vi "Gantry_motion.vi"() -> ()   [LabVIEW 2016]
uses:
  Classes/Controllers/Motion/Copy of A3200 Folder/A3200.lvclass
  D:/INTT/V1/Classes/Controllers/Motion/Copy of Motion Folder/Motion.lvclass
  Classes/Controllers/Motion/Copy of Motion Folder/Motion.lvclass
panel:
  out "millisecond timer value":u32
  in  "Stop":bool
  in  "Z Speed":dbl=5.0 format="%#_13g"
  in  "Z":dbl=10.0 format="%#_13g"
  out "Gantry position":dbl[](array[numeric])
  in  "Speed":dbl=20.0
  in  "XY":dbl[](array[numeric])
  out "number of tasks excuted":i32
  in  "Z GO":bool
  in  "XY GO":bool
  in  "XYZ GO":bool
  in  "XYZTheta In":dbl[](array[numeric])=[600.0, 600.0, 0.0, 0.0]
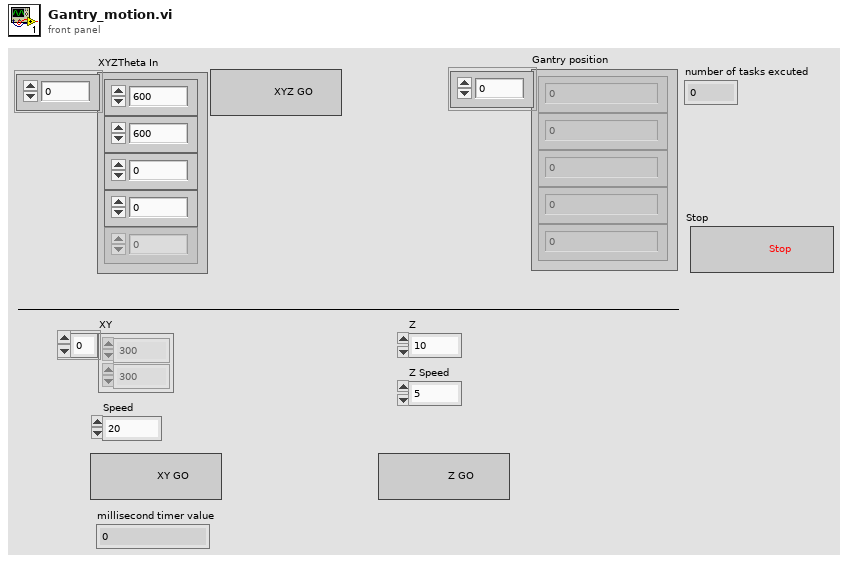
[diagram p1: front panel]
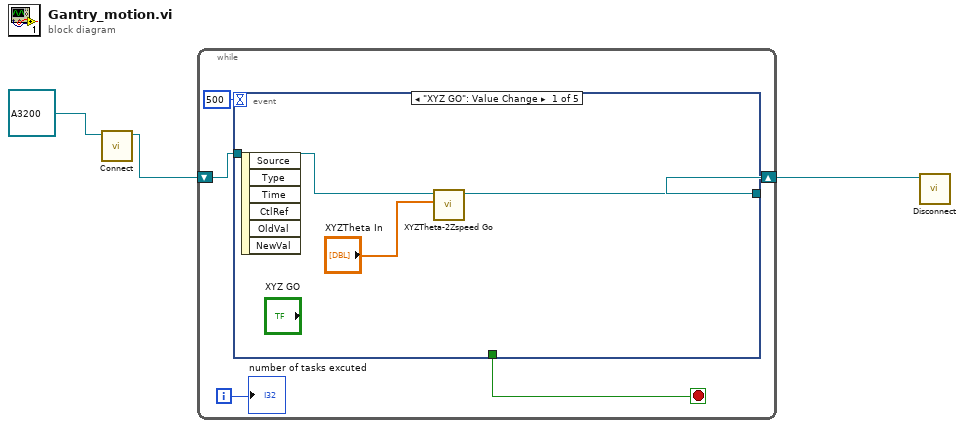
[diagram p0: block diagram]
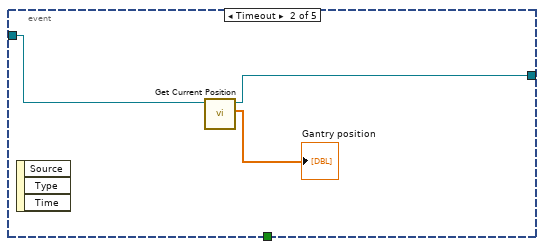
[diagram p2: hidden frame]
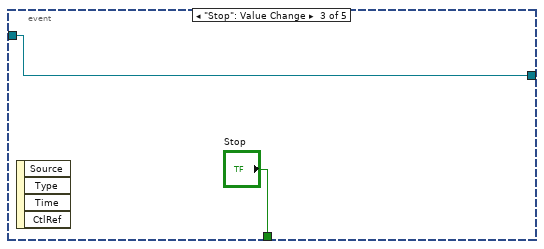
[diagram p3: hidden frame]
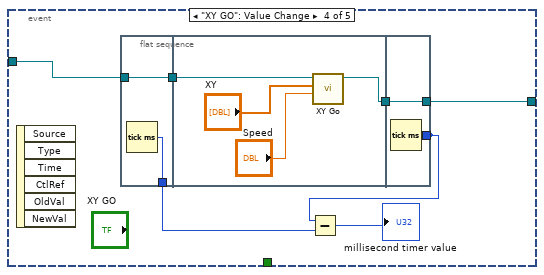
[diagram p4: hidden frame]
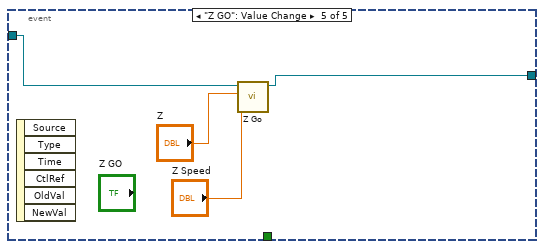
[diagram p5: hidden frame]
diagram:
  n1 = call-dynamic "Connect.vi"("Gantry in"=refnum<class "A3200.lvclass"> refnum ("A3200.lvclass")) -> ("Gantry out"=w1:refnum<class "A3200.lvclass">)  [unwired: 9 in, 1 out]
  n2 = while {
    shift-right: [w7] -> w2
    shift-left: w1 -> [w8]
    i -> [w6]
    stop <- w4 stop-if-true
    n3 = event shown="[0] \"XYZ GO\": Value Change" {
      selector: _ -> [_ _ _ _ _]
      dyn-events: _ -> [_ _ _ _ _]
      timeout: 500 -> [_ _ _ _ _]
      tunnel: w8 -> [w11 w14 w15 w23 w35]
      tunnel: [w10 w12 w15 w22 w32] -> w7
      tunnel: [_ _ "Stop" _ _] -> w4
      event "XYZ GO": Value Change {
        n4 = event-data() -> ()  [unwired: 1 in, 6 out]
        n5 = call "XYZTheta-2Zspeed Go.vi"("XYZTheta In"="XYZTheta In", "Motion in"=w11) -> ("Motion out"=w10:refnum<class "A3200.lvclass">)  [unwired: 7 in, 2 out]
      }
      event Timeout {
        n6 = event-data() -> ()  [unwired: 1 in, 3 out]
        n7 = call-dynamic "Get Current Position.vi"("Gantry in"=w14) -> ("XYZTheta Out"=→"Gantry position":dbl[], "Gantry out"=w12:refnum<class "A3200.lvclass">)  [unwired: 8 in, 1 out]
      }
      event "Stop": Value Change {
        n8 = event-data() -> ()  [unwired: 1 in, 4 out]
      }
      event "XY GO": Value Change {
        n9 = event-data() -> ()  [unwired: 1 in, 6 out]
        n10 = flat-sequence {
          tunnel: w23 -> [w25]
          tunnel: [w25] -> w21
          tunnel: [w24] -> w18
          tunnel: w21 -> [w29]
          tunnel: [w28] -> w20
          tunnel: [w31] -> w22
          tunnel: w20 -> [w31]
          tunnel: [w30] -> _
          tunnel: [w30] -> w19
          frame #0 {
            n11 = Tick Count (ms)() -> (millisecond timer value=w24:u32)
          }
          frame #1 {
            n12 = call-dynamic "XY Go.vi"("Speed"="Speed", "XY"="XY", "Gantry in"=w29) -> ("Gantry out"=w28:refnum<class "A3200.lvclass">)  [unwired: 7 in, 1 out]
          }
          frame #2 {
            n13 = Tick Count (ms)() -> (millisecond timer value=w30:u32)
          }
        }
        n14 = Subtract(x=w19, y=w18) -> (x-y=→"millisecond timer value":u32)
      }
      event "Z GO": Value Change {
        n15 = event-data() -> ()  [unwired: 1 in, 6 out]
        n16 = call-dynamic "Z Go.vi"("Speed"="Z Speed", "Position"="Z", "Gantry in"=w35) -> ("Gantry out"=w32:refnum<class "A3200.lvclass">)  [unwired: 7 in, 1 out]
      }
    }
    "number of tasks excuted" <- w6
  }
  n17 = call-dynamic "Disconnect.vi"("Gantry in"=w2) -> ()  [unwired: 9 in, 1 out]
